vi "Set Open Time.vi"(8 "error in (no error)":errorcluster, 10 "Open time (ms)":i32, 11 "hdl":i32) -> (0 "error out":errorcluster, 3 "hdl out":i32)   [LabVIEW 2013, in "Thorlabs_SC10.lvlib"]
doc: "Returns current NTC10K sensor Beta value."
uses:
  <instrlib>/Thorlabs_SC10/Thorlabs_SC10.lvlib
  <instrlib>/Thorlabs_SC10/Data/SC10CommandLib_x64.dll
  <instrlib>/Thorlabs_SC10/Data/SC10CommandLib_win32.dll
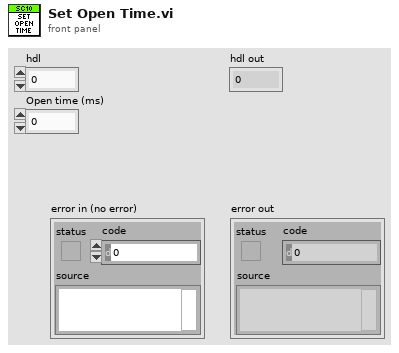
[diagram p1: front panel]
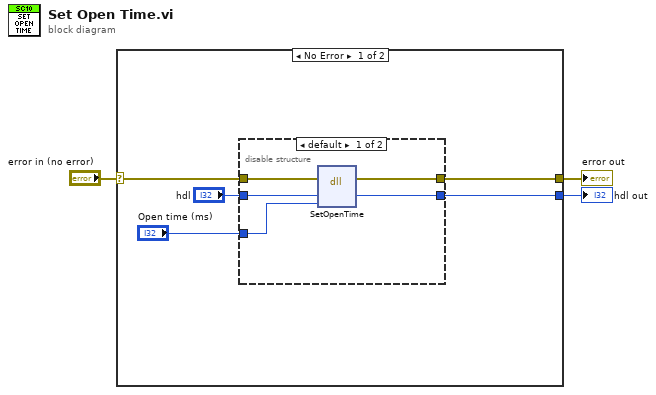
[diagram p0: block diagram]
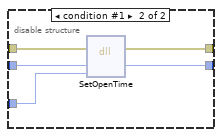
[diagram p2: hidden frame]
diagram:
  n1 = case shown="No Error" "error in (no error)" {
    selector: "error in (no error)" -> [w8 w19]
    tunnel: [w7 w19] -> w3
    tunnel: [w6 _] -> w1
    frame No Error {
      n2 = disable-structure shown="default" {
        disable-tunnel: w8 -> [w13 w18]
        disable-tunnel: [w12 w17] -> w7
        disable-tunnel: [w11 w16] -> w6
        disable-tunnel: "hdl" -> [w10 w15]
        disable-tunnel: "Open time (ms)" -> [w9 w14]
        frame condition #0 (active) {
          n3 = dll-call lib="C:/Program Files (x86)/National Instruments/LabVIEW 2013/instr.lib/Thorlabs_SC10/Data/SC10CommandLib_win32.dll" fn="SetOpenTime"(error in=w13, "hdl"=w10, "value"=w9) -> (error out=w12:errorcluster, "hdl"=w11:i32)  [unwired: 4 in, 1 out]
        }
        frame condition #1 {
          n4 = dll-call lib="C:/Program Files/National Instruments/LabVIEW 2013/instr.lib/Thorlabs_SC10/Data/SC10CommandLib_x64.dll" fn="SetOpenTime"(error in=w18, "hdl"=w15, "value"=w14) -> (error out=w17:errorcluster, "hdl"=w16:i32)  [unwired: 4 in, 1 out]
        }
      }
    }
    frame Error {
    }
  }
  "error out" <- w3
  "hdl out" <- w1
